vi "filter release date.vi"(8 "error in (no error)":errorcluster, 10 "Release Week":timestamp, 11 "manager_daemon in":refnum<class "manager_daemon.lvclass">) -> (0 "error out":errorcluster, 3 "manager_daemon out":refnum<class "manager_daemon.lvclass">)   [LabVIEW 2024, in "manager_daemon.lvclass"]
uses:
  manager_daemon.lvclass
  manager_daemon.lvclass/manager_daemon.ctl
  type_defs/cmd--enum.ctl
  type_defs/msg--cluster.ctl
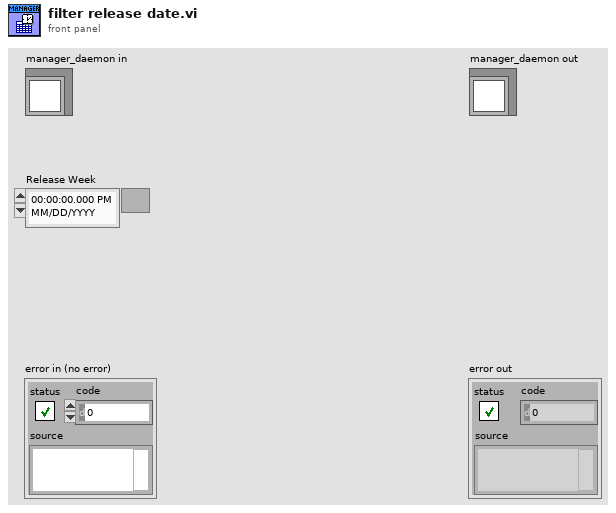
[diagram p1: front panel]
types:
  T1 = typedef "manager_daemon.lvclass/cmd--enum.ctl" = enum16{"init", "run", "load binaries", "build binaries", "save binaries", "updated volume", "return vol path by id", "display info", "filter release week", "apply filter", "add volume", "add issues", "add issue", "delete volume", "delete issues", "exit"}
  T2 = typedef "manager_daemon.lvclass/msg--cluster.ctl" = cluster{"cmd":T1, "data":variant}
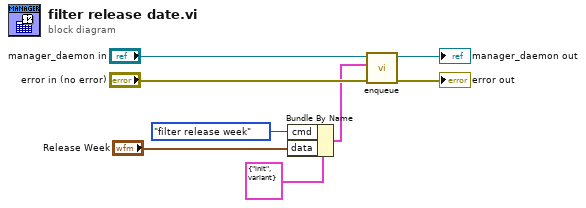
[diagram p0: block diagram]
diagram:
  n1 = Bundle By Name(cluster=T2 {"cmd"=enum."init", "data"=variant} ("msg"), "cmd"=cmd--enum."filter release week", "data"="Release Week") -> (w1:T2)
  n2 = call "enqueue.vi"("error in (no error)"="error in (no error)", "msg"=w1, "manager_daemon in"="manager_daemon in") -> ("error out"=→"error out":errorcluster, "manager_daemon out"=→"manager_daemon out":refnum<class "manager_daemon.lvclass">)  [unwired: 7 in]
